vi "Refresh.vi"(8 "error in (no error)":errorcluster, 11 "ArrayManager in":refnum<class "ArrayManager.lvclass">) -> (0 "error out":errorcluster, 3 "ArrayManager out":refnum<class "ArrayManager.lvclass">)   [LabVIEW 2020, in "OOPanel.lvlib" / "ArrayManager.lvclass"]
uses:
  <vilib>/IlluminatedG/IG OOPanel/OOPanel/ArrayManager/ArrayManager.lvclass
  <vilib>/IlluminatedG/IG OOPanel/OOPanel/ArrayManager/ArrayManager.lvclass/ArrayManager.ctl
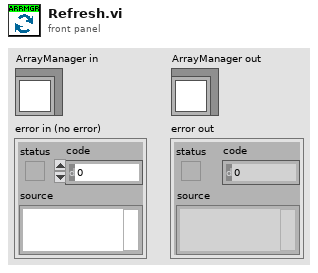
[diagram p1: front panel]
types:
  T1 = typedef "OOPanel.lvlib/ArrayManager.lvclass/Event Regs.ctl" = cluster{"Event Reg":refnum<event-registration>, "Last Update Ticks ms":u32}
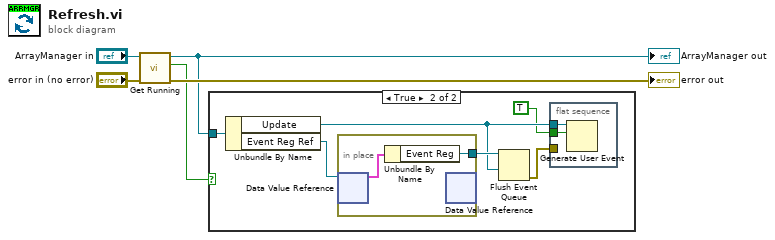
[diagram p0: block diagram]
diagram:
  n1 = call <vilib>:"Get Running.vi"("error in (no error)"="error in (no error)", "ArrayManager in"="ArrayManager in") -> ("error out"=→"error out":errorcluster, "Running"=w2:bool, "ArrayManager out"=w1:refnum<class "ArrayManager.lvclass">)  [unwired: 7 in]
  "ArrayManager out" <- w1
  n2 = case shown="True" w2 {
    tunnel: w1 -> [_ w11]
    frame False {
    }
    frame True {
      n3 = Unbundle By Name(w11) -> ("Update"=w8:refnum<user-event>, "Event Reg Ref"=w10:refnum<data-value>)
      n4 = in-place {
        in-place-border: [w14] -> w9
        n5 = in-place-dvr #1(w10) -> (w15:T1)  [unwired: 1 out]
        n6 = Unbundle By Name(w15) -> ("Event Reg"=w14:refnum<event-registration>)
        n7 = in-place-dvr #1() -> ()  [unwired: 1 in, 2 out]
      }
      n8 = Flush Event Queue(0:w9, 2:w8) -> (11:w6:errorcluster)  [unwired: 4 in, 2 out]
      n9 = flat-sequence {
        tunnel: w8 -> [w13]
        tunnel: TRUE ("event data") -> [w12]
        tunnel: w6 -> [_]
        frame #0 {
          n10 = Generate User Event(user event=w13, event data cluster=w12) -> ()  [unwired: 2 in, 2 out]
        }
      }
    }
  }
